vi "Check Encoders (Debug).vi"() -> ()   [LabVIEW 2009]
panel:
  out "Debug":string
  out "MC Init Complete":bool=TRUE
  in  "MC VISA resource in":refnum<visa-resource-name>="ASRL1::INSTR"
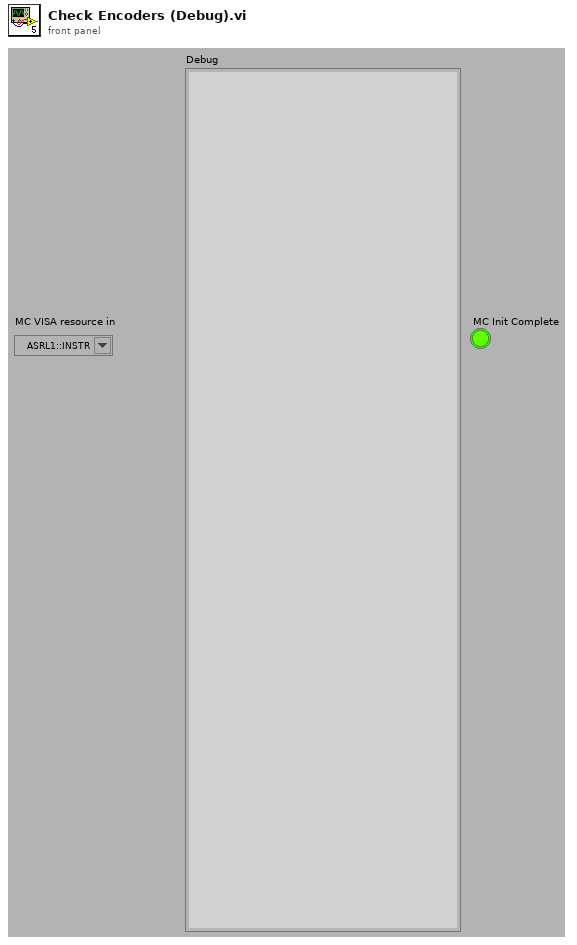
[diagram p1: front panel]
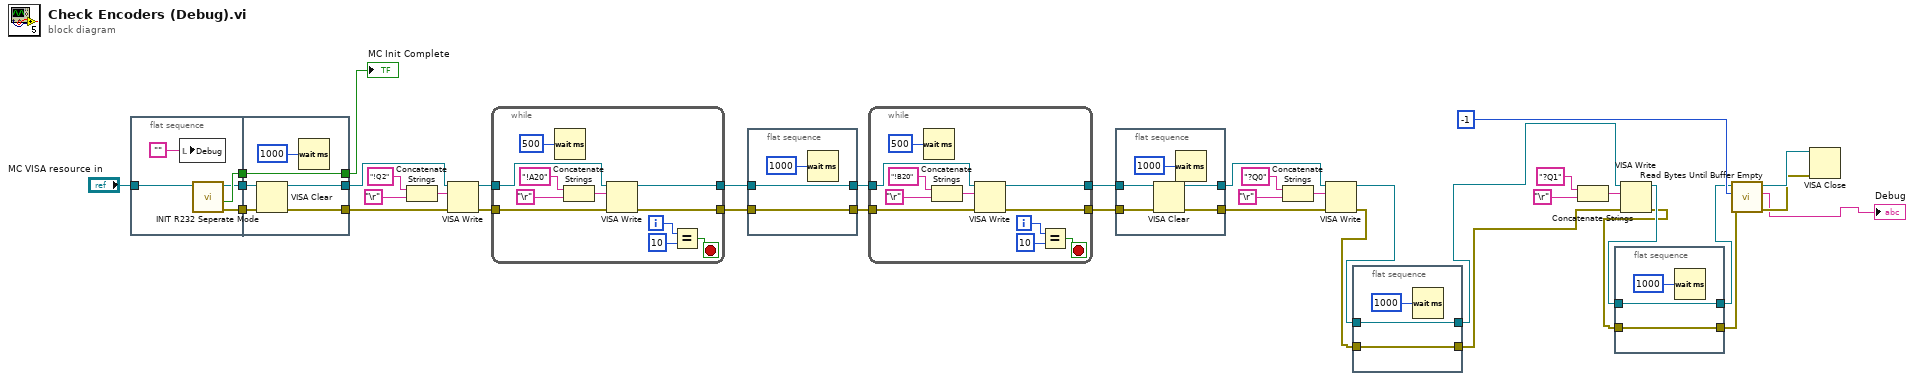
[diagram p0: block diagram]
diagram:
  n1 = flat-sequence {
    tunnel: "MC VISA resource in" -> [w43]
    tunnel: [w42] -> w34
    tunnel: [w41] -> w33
    tunnel: [w40] -> w32
    tunnel: [w44] -> w35
    tunnel: [w45] -> w36
    tunnel: [w49] -> w37
    tunnel: w34 -> [w49]
    tunnel: w33 -> [w46]
    tunnel: w32 -> [w47]
    frame #0 {
      n2 = local write "Debug"("") -> ()
      n3 = call "INIT R232 Seperate Mode.vi"("MC VISA resource in"=w43) -> ("MC error out"=w40:errorcluster, "MC Init Complete"=w42:bool, "MC VISA resource  out"=w41:refnum<visa-resource-name>)  [unwired: 8 in]
    }
    frame #1 {
      n4 = VISA Clear(VISA resource name=w46, error in (no error)=w47) -> (VISA resource name out=w45:refnum<visa-resource-name>, error out=w44:errorcluster)
      n5 = Wait (ms)(milliseconds to wait=u32 1000) -> ()  [unwired: 1 out]
    }
  }
  n6 = Concatenate Strings("!Q2" ("write buffer"), "\r") -> (w29:string)
  n7 = VISA Write(VISA resource name=w36, write buffer=w29, error in (no error)=w35) -> (VISA resource name out=w20:refnum<visa-resource-name>, error out=w19:errorcluster)  [unwired: 1 out]
  n8 = while {
    tunnel: w20 -> [w54]
    tunnel: w19 -> [w53]
    tunnel: [w52] -> w23
    tunnel: [w51] -> w21
    i -> [w60]
    stop <- w58 stop-if-true
    n9 = Wait (ms)(milliseconds to wait=u32 500) -> ()  [unwired: 1 out]
    n10 = Concatenate Strings("!A20" ("write buffer"), "\r") -> (w57:string)
    n11 = VISA Write(VISA resource name=w54, write buffer=w57, error in (no error)=w53) -> (VISA resource name out=w52:refnum<visa-resource-name>, error out=w51:errorcluster)  [unwired: 1 out]
    n12 = Equal?(x=w60, y=10) -> (x = y?=w58:bool)
  }
  n13 = flat-sequence {
    tunnel: [w62] -> w18
    tunnel: w23 -> [w62]
    tunnel: [w61] -> w22
    tunnel: w21 -> [w61]
    frame #0 {
      n14 = Wait (ms)(milliseconds to wait=u32 1000) -> ()  [unwired: 1 out]
    }
  }
  n15 = while {
    tunnel: w22 -> [w68]
    tunnel: [w67] -> w25
    tunnel: [w66] -> w24
    tunnel: w18 -> [w65]
    i -> [w74]
    stop <- w72 stop-if-true
    n16 = Wait (ms)(milliseconds to wait=u32 500) -> ()  [unwired: 1 out]
    n17 = Concatenate Strings("!B20" ("write buffer"), "\r") -> (w71:string)
    n18 = VISA Write(VISA resource name=w65, write buffer=w71, error in (no error)=w68) -> (VISA resource name out=w67:refnum<visa-resource-name>, error out=w66:errorcluster)  [unwired: 1 out]
    n19 = Equal?(x=w74, y=10) -> (x = y?=w72:bool)
  }
  n20 = flat-sequence {
    tunnel: [w77] -> w10
    tunnel: w25 -> [w78]
    tunnel: [w75] -> w9
    tunnel: w24 -> [w76]
    frame #0 {
      n21 = VISA Clear(VISA resource name=w78, error in (no error)=w76) -> (VISA resource name out=w77:refnum<visa-resource-name>, error out=w75:errorcluster)
      n22 = Wait (ms)(milliseconds to wait=u32 1000) -> ()  [unwired: 1 out]
    }
  }
  n23 = Concatenate Strings("?Q0" ("write buffer"), "\r") -> (w26:string)
  n24 = VISA Write(VISA resource name=w10, write buffer=w26, error in (no error)=w9) -> (VISA resource name out=w3:refnum<visa-resource-name>, error out=w4:errorcluster)  [unwired: 1 out]
  n25 = flat-sequence {
    tunnel: [w81] -> w1
    tunnel: w3 -> [w81]
    tunnel: [w80] -> w2
    tunnel: w4 -> [w80]
    frame #0 {
      n26 = Wait (ms)(milliseconds to wait=u32 1000) -> ()  [unwired: 1 out]
    }
  }
  n27 = Concatenate Strings("?Q1" ("write buffer"), "\r") -> (w15:string)
  n28 = flat-sequence {
    tunnel: [w84] -> w5
    tunnel: w8 -> [w84]
    tunnel: [w83] -> w6
    tunnel: w7 -> [w83]
    frame #0 {
      n29 = Wait (ms)(milliseconds to wait=u32 1000) -> ()  [unwired: 1 out]
    }
  }
  n30 = VISA Write(VISA resource name=w1, write buffer=w15, error in (no error)=w2) -> (VISA resource name out=w8:refnum<visa-resource-name>, error out=w7:errorcluster)  [unwired: 1 out]
  n31 = call "Read Bytes Until Buffer Empty.vi"("error in"=w6, "timeout (ms)"=-1, "MC VISA resource in"=w5) -> ("error out"=w12:errorcluster, "read buffer"=→"Debug":string, "MC VISA resource  out"=w13:refnum<visa-resource-name>)  [unwired: 6 in]
  n32 = VISA Close(VISA resource name=w13, error in (no error)=w12) -> ()  [unwired: 1 out]
  "MC Init Complete" <- w37
